vi "SentinelController v33.vi"() -> ()   [LabVIEW 2011] (continued)
                                n2600 = local write "NS6040 tester states H1 hid"(SC_NS6040_tester_states."sending Fullsites?" ("NS6040 tester states H1 hid")) -> ()
                                }
                                frame True {
                                n2601 = flat-sequence {
                                frame #0 {
                                n2602 = while {
                                stop <- w1021 stop-if-true
                                n2603 = Wait (ms)(milliseconds to wait=u32 100) -> ()  [unwired: 1 out]
                                n2604 = One Button Dialog(message="Read error while reading FR?,\nclosing Bus and re-initializing" ("Reply from Sentinel Controller to tester")) -> (true=w1021:bool)  [unwired: 1 in]
                                }
                                }
                                frame #1 {
                                n2605 = local read "VISA bus 1 resource name out hid"() -> (w1027:refnum<visa-resource-name>)
                                n2606 = local read "VISA bus 1 error out hid"() -> (w1026:errorcluster)
                                n2607 = VISA Close(VISA resource name=w1027, error in (no error)=w1026) -> (error out=w1025:errorcluster)
                                n2608 = Unbundle By Name(w1025) -> ("status"=w1024:bool)
                                n2609 = local write "VISA bus 1 close error"(w1024) -> ()
                                }
                                frame #2 {
                                n2610 = local write "VISA bus 1 close error"(FALSE ("H1 online")) -> ()
                                n2611 = local write "NS6040 tester states H1 hid"(SC_NS6040_tester_states."initializing bus" ("NS6040 tester states H1 hid")) -> ()
                                }
                                }
                                }
                                }
                                }
                                frame "sending Fullsites?" {
                                n2612 = flat-sequence {
                                frame #0 {
                                n2613 = flat-sequence {
                                tunnel: [w1035] -> w1032
                                tunnel: [w1034] -> w1030
                                tunnel: [w1041] -> w1033
                                tunnel: w1032 -> [w1041]
                                tunnel: [w1040] -> w1031
                                tunnel: w1030 -> [w1040]
                                tunnel: w1033 -> [w1044]
                                tunnel: w1031 -> [w1043]
                                frame #0 {
                                w1036 = "Fullsites?\n"
                                n2614 = local read "VISA bus 1 resource name out hid"() -> (w1038:refnum<visa-resource-name>)
                                n2615 = local read "VISA bus 1 error out hid"() -> (w1037:errorcluster)
                                n2616 = local write "GPIB bus 1 traffic"(w1036) -> ()
                                n2617 = VISA Write(VISA resource name=w1038, write buffer=w1036, error in (no error)=w1037) -> (VISA resource name out=w1034:refnum<visa-resource-name>, error out=w1035:errorcluster)  [unwired: 1 out]
                                n2618 = Unbundle By Name(w1035) -> ("status"=w1039:bool)
                                n2619 = local write "GPIB bus 1 write error"(w1039) -> ()
                                }
                                frame #1 {
                                n2620 = Wait (ms)(milliseconds to wait=u32 2) -> ()  [unwired: 1 out]
                                }
                                frame #2 {
                                n2621 = local read "GPIB bus 1 traffic"() -> (w1051:string)
                                n2622 = VISA Read(VISA resource name=w1043, byte count=u32 256, error in (no error)=w1044) -> (VISA resource name out=w1046:refnum<visa-resource-name>, read buffer=w1052:string, error out=w1047:errorcluster)  [unwired: 1 out]
                                n2623 = local write "VISA bus 1 resource name out hid"(w1046) -> ()
                                n2624 = local write "H1 FULLSITES? response hid"(w1052) -> ()
                                n2625 = Unbundle By Name(w1047) -> ("status"=w1053:bool)
                                n2626 = Concatenate Strings(w1051, "\r\n", "Bus 1 read: " ("string"), w1052) -> (w1049:string)
                                n2627 = local write "GPIB bus 1 read error"(w1053) -> ()
                                n2628 = local write "GPIB bus 1 traffic"(w1049) -> ()
                                }
                                }
                                }
                                frame #1 {
                                n2629 = local read "GPIB bus 1 read error"() -> (w1054:bool)
                                n2630 = case shown="False" w1054 {
                                frame False {
                                n2631 = flat-sequence {
                                frame #0 {
                                w1063 = "%032b"  # format string
                                n2632 = local read "H1 FULLSITES? response hid"() -> (w1056:string)
                                n2633 = call <vilib>:"Space Constant.vi"() -> ("String"=w1058:string)
                                n2634 = Concatenate Strings("Fullsites" ("regular expression"), w1058) -> (w1057:string)
                                n2635 = call <vilib>:"Trim Whitespace.vi"("string"=w1056) -> ("trimmed string"=w1055:string)  [unwired: 1 in]
                                n2636 = Match Pattern(string=w1055, regular expression=w1057) -> (after substring=w1061:string)  [unwired: 1 in, 3 out]
                                n2637 = Hexadecimal String To Number(string=w1061, default (0uL)=u64 0 ("default (0 U32)")) -> (number=w1064:u64)  [unwired: 1 in, 1 out]
                                n2638 = Format Into String "Format Into String"(format string=w1063, w1064) -> (resulting string=w1060:string)  [unwired: 2 in, 1 out]
                                n2639 = local write "H1 FULLSITES? binary hid"(w1060) -> ()
                                }
                                frame #1 {
                                n2640 = Tick Count (ms)() -> (millisecond timer value=w1068:u32)
                                n2641 = Tick Count (ms)() -> (millisecond timer value=w1067:u32)
                                n2642 = local write "H1 wt start hidden"(w1068) -> ()
                                n2643 = local write "H1 it end hidden"(w1067) -> ()
                                n2644 = local write "H1 Indexing"(FALSE ("h1 indexing")) -> ()
                                n2645 = local write "H1 Testing"(FALSE ("h1 indexing")) -> ()
                                }
                                frame #2 {
                                n2646 = local read "H1 it start hidden"() -> (w1072:u32)
                                n2647 = local read "H1 it end hidden"() -> (w1073:u32)
                                n2648 = Subtract(x=w1073, y=w1072) -> (x-y=w1069:u32)
                                n2649 = Divide(x=w1069, y=u32 1000) -> (x/y=w1071:dbl)
                                n2650 = local write "H1 measured Index Time"(w1071) -> ()
                                }
                                frame #3 {
                                n2651 = local write "NS6040 tester states H1 hid"(SC_NS6040_tester_states."testing" ("NS6040 tester states H1 hid")) -> ()
                                }
                                }
                                }
                                frame True {
                                n2652 = flat-sequence {
                                frame #0 {
                                n2653 = while {
                                stop <- w1075 stop-if-true
                                n2654 = Wait (ms)(milliseconds to wait=u32 100) -> ()  [unwired: 1 out]
                                n2655 = One Button Dialog(message="Read error while reading FULLSITES?,\nclosing Bus and re-initializing" ("Reply from Sentinel Controller to tester")) -> (true=w1075:bool)  [unwired: 1 in]
                                }
                                }
                                frame #1 {
                                n2656 = local read "VISA bus 1 resource name out hid"() -> (w1081:refnum<visa-resource-name>)
                                n2657 = local read "VISA bus 1 error out hid"() -> (w1080:errorcluster)
                                n2658 = VISA Close(VISA resource name=w1081, error in (no error)=w1080) -> (error out=w1079:errorcluster)
                                n2659 = Unbundle By Name(w1079) -> ("status"=w1078:bool)
                                n2660 = local write "VISA bus 1 close error"(w1078) -> ()
                                }
                                frame #2 {
                                n2661 = local write "VISA bus 1 close error"(FALSE ("H1 online")) -> ()
                                n2662 = local write "NS6040 tester states H1 hid"(SC_NS6040_tester_states."initializing bus" ("NS6040 tester states H1 hid")) -> ()
                                }
                                }
                                }
                                }
                                }
                                }
                                }
                                frame "testing" {
                                n2663 = flat-sequence {
                                frame #0 {
                                n2664 = while {
                                stop <- w1084 stop-if-true
                                n2665 = local read "H1 Lock"() -> (w1084:bool)
                                n2666 = Wait (ms)(milliseconds to wait=u32 1) -> ()  [unwired: 1 out]
                                }
                                }
                                frame #1 {
                                n2667 = local write "H1 Ready with sites"(FALSE ("H1 Waiting")) -> ()
                                n2668 = Tick Count (ms)() -> (millisecond timer value=w1095:u32)
                                n2669 = Tick Count (ms)() -> (millisecond timer value=w1094:u32)
                                n2670 = local write "H1 Testing"(TRUE ("testing")) -> ()
                                n2671 = local write "H1 Indexing"(FALSE ("waiting")) -> ()
                                n2672 = local write "H1 wt end hidden"(w1095) -> ()
                                n2673 = local write "H1 tt start hidden"(w1094) -> ()
                                n2674 = local read "GPIB bus 1 traffic"() -> (w1087:string)
                                n2675 = Concatenate Strings(w1087, "\r\n", "Bus 1: " ("string"), "testing" ("string")) -> (w1089:string)
                                n2676 = local write "GPIB bus 1 traffic"(w1089) -> ()
                                }
                                frame #2 {
                                n2677 = local read "H1 wt start hidden"() -> (w1099:u32)
                                n2678 = local read "H1 wt end hidden"() -> (w1100:u32)
                                n2679 = Subtract(x=w1100, y=w1099) -> (x-y=w1098:u32)
                                n2680 = Divide(x=w1098, y=u32 1000) -> (x/y=w1096:dbl)
                                n2681 = local write "H1 measured Wait Time"(w1096) -> ()
                                }
                                frame #3 {
                                n2682 = local write "NS6040 tester states H1 hid"(SC_NS6040_tester_states."sending BINON?" ("NS6040 tester states H1 hid")) -> ()
                                }
                                }
                                }
                                frame "sending BINON?" {
                                n2683 = flat-sequence {
                                tunnel: [w1110] -> w1104
                                tunnel: [w1109] -> w1103
                                tunnel: w1104 -> [w1120]
                                tunnel: w1103 -> [w1119]
                                tunnel: [w1118] -> w1102
                                tunnel: w1102 -> [w1137]
                                frame #0 {
                                n2684 = while {
                                stop <- w1106 continue-if-true
                                n2685 = local read "H1 Lock"() -> (w1106:bool)
                                n2686 = Wait (ms)(milliseconds to wait=u32 1) -> ()  [unwired: 1 out]
                                }
                                }
                                frame #1 {
                                n2687 = local read "Binning string from tester hid"() -> (w1107:string)
                                n2688 = local write "H1 binning string hid"(w1107) -> ()
                                }
                                frame #2 {
                                n2689 = local read "VISA bus 1 resource name out hid"() -> (w1116:refnum<visa-resource-name>)
                                n2690 = local read "VISA bus 1 error out hid"() -> (w1117:errorcluster)
                                n2691 = local read "H1 binning string hid"() -> (w1108:string)
                                n2692 = local read "GPIB bus 1 traffic"() -> (w1114:string)
                                n2693 = VISA Write(VISA resource name=w1116, write buffer=w1108, error in (no error)=w1117) -> (VISA resource name out=w1109:refnum<visa-resource-name>, error out=w1110:errorcluster)  [unwired: 1 out]
                                n2694 = local write "VISA bus 1 error out hid"(w1110) -> ()
                                n2695 = Unbundle By Name(w1110) -> ("status"=w1115:bool)
                                n2696 = Concatenate Strings(w1114, "\r\n", "Bus 1 write: " ("string"), w1108) -> (w1112:string)
                                n2697 = local write "GPIB bus 1 traffic"(w1112) -> ()
                                n2698 = local write "GPIB bus 1 write error"(w1115) -> ()
                                }
                                frame #3 {
                                n2699 = while {
                                tunnel: w1120 -> [w1127]
                                tunnel: w1119 -> [w1126]
                                tunnel: [w1121] -> w1118
                                stop <- w1123 stop-if-true
                                n2700 = local read "GPIB bus 1 traffic"() -> (w1129:string)
                                n2701 = VISA Read(VISA resource name=w1126, byte count=u32 256, error in (no error)=w1127) -> (VISA resource name out=w1134:refnum<visa-resource-name>, read buffer=w1121:string, error out=w1133:errorcluster)  [unwired: 1 out]
                                n2702 = local write "VISA bus 1 resource name out hid"(w1134) -> ()
                                n2703 = Unbundle By Name(w1133) -> ("status"=w1128:bool)
                                n2704 = Match True/False String(2:"false string" ("false string"), 3:"ECHO:", 4:w1121) -> (0:w1123:bool)  [unwired: 1 out]
                                n2705 = local write "GPIB bus 1 read error"(w1128) -> ()
                                n2706 = Concatenate Strings(w1129, "\r\n", "Bus 1 read: " ("string"), w1121) -> (w1131:string)
                                n2707 = local write "GPIB bus 1 traffic"(w1131) -> ()
                                n2708 = Wait (ms)(milliseconds to wait=u32 5) -> ()  [unwired: 1 out]
                                }
                                }
                                frame #4 {
                                n2709 = local read "GPIB bus 1 read error"() -> (w1136:bool)
                                n2710 = case shown="False" w1136 {
                                tunnel: w1137 -> [w1138 _]
                                frame False {
                                n2711 = local write "H1 echo hid"(w1138) -> ()
                                n2712 = local read "H1 binning string hid"() -> (w1139:string)
                                n2713 = Equal?(x=w1138, y=w1139) -> (x = y?=w1140:bool)
                                n2714 = case shown="True" w1140 {
                                frame False {
                                n2715 = local write "NS6040 tester states H1 hid"(SC_NS6040_tester_states."sending ECHONG" ("NS6040 tester states H1 hid")) -> ()
                                }
                                frame True {
                                n2716 = local write "NS6040 tester states H1 hid"(SC_NS6040_tester_states."sending ECHOOK" ("NS6040 tester states H1 hid")) -> ()
                                }
                                }
                                }
                                frame True {
                                n2717 = flat-sequence {
                                frame #0 {
                                n2718 = while {
                                stop <- w1144 stop-if-true
                                n2719 = Wait (ms)(milliseconds to wait=u32 100) -> ()  [unwired: 1 out]
                                n2720 = One Button Dialog(message="Echo readback error for H1.\nClosing Bus 1.", button name ("OK")="Dismiss") -> (true=w1144:bool)
                                }
                                }
                                frame #1 {
                                n2721 = local write "NS6040 tester states H1 hid"(SC_NS6040_tester_states."closing bus" ("NS6040 tester states H1 hid")) -> ()
                                }
                                }
                                }
                                }
                                }
                                }
                                }
                                frame "sending ECHONG" {
                                n2722 = flat-sequence {
                                frame #0 {
                                w1148 = "ECHONG\n"
                                n2723 = local read "VISA bus 1 resource name out hid"() -> (w1155:refnum<visa-resource-name>)
                                n2724 = local read "VISA bus 1 error out hid"() -> (w1156:errorcluster)
                                n2725 = local read "GPIB bus 1 traffic"() -> (w1153:string)
                                n2726 = VISA Write(VISA resource name=w1155, write buffer=w1148, error in (no error)=w1156) -> (error out=w1149:errorcluster)  [unwired: 2 out]
                                n2727 = Unbundle By Name(w1149) -> ("status"=w1154:bool)
                                n2728 = Concatenate Strings(w1153, "\r\n", "Bus 1 write: " ("string"), w1148) -> (w1151:string)
                                n2729 = local write "VISA bus 1 error out hid"(w1149) -> ()
                                n2730 = local write "GPIB bus 1 traffic"(w1151) -> ()
                                n2731 = local write "GPIB bus 1 write error"(w1154) -> ()
                                }
                                frame #1 {
                                n2732 = while {
                                stop <- w1157 stop-if-true
                                n2733 = Wait (ms)(milliseconds to wait=u32 100) -> ()  [unwired: 1 out]
                                n2734 = One Button Dialog(message="ECHO from handler 1 did not match BINON'\nError message from \"sending ECHONG\" state\nBINON message will be resent.") -> (true=w1157:bool)  [unwired: 1 in]
                                }
                                }
                                frame #2 {
                                n2735 = local write "NS6040 tester states H1 hid"(SC_NS6040_tester_states."sending BINON?" ("NS6040 tester states H1 hid")) -> ()
                                }
                                }
                                }
                                frame "sending ECHOOK" {
                                n2736 = flat-sequence {
                                frame #0 {
                                w1161 = "ECHOOK\n"
                                n2737 = local read "VISA bus 1 resource name out hid"() -> (w1168:refnum<visa-resource-name>)
                                n2738 = local read "VISA bus 1 error out hid"() -> (w1169:errorcluster)
                                n2739 = local read "GPIB bus 1 traffic"() -> (w1166:string)
                                n2740 = VISA Write(VISA resource name=w1168, write buffer=w1161, error in (no error)=w1169) -> (error out=w1162:errorcluster)  [unwired: 2 out]
                                n2741 = Unbundle By Name(w1162) -> ("status"=w1167:bool)
                                n2742 = Concatenate Strings(w1166, "\r\n", "Bus 1 write: " ("string"), w1161) -> (w1164:string)
                                n2743 = local write "VISA bus 1 error out hid"(w1162) -> ()
                                n2744 = local write "GPIB bus 1 traffic"(w1164) -> ()
                                n2745 = local write "GPIB bus 1 write error"(w1167) -> ()
                                }
                                frame #1 {
                                n2746 = Tick Count (ms)() -> (millisecond timer value=w1171:u32)
                                n2747 = Tick Count (ms)() -> (millisecond timer value=w1172:u32)
                                n2748 = local write "H1 Ready with sites"(FALSE ("waiting")) -> ()
                                n2749 = local write "H1 Testing"(FALSE ("waiting")) -> ()
                                n2750 = local write "H1 Indexing"(TRUE ("waiting")) -> ()
                                n2751 = local write "H1 tt end hidden"(w1171) -> ()
                                n2752 = local write "H1 it start hidden"(w1172) -> ()
                                }
                                frame #2 {
                                n2753 = local read "H1 tt start hidden"() -> (w1178:u32)
                                n2754 = local read "H1 tt end hidden"() -> (w1179:u32)
                                n2755 = Subtract(x=w1179, y=w1178) -> (x-y=w1177:u32)
                                n2756 = Divide(x=w1177, y=u32 1000) -> (x/y=w1175:dbl)
                                n2757 = local write "H1 measured Test Time"(w1175) -> ()
                                }
                                frame #3 {
                                n2758 = local read "H1 binning string hid"() -> (w1180:string)
                                n2759 = local read "H1 FULLSITES? binary hid"() -> (w1196:string)
                                n2760 = String Subset(string=w1180, offset (0)=6, length (rest)=35 ("length (rest)")) -> (substring=w1192:string)
                                n2761 = local read "H1 Device Count"() -> (w1181:u32)
                                n2762 = local read "H1 Good Units"() -> (w1182:u32)
                                n2763 = Search and Replace String(replace all?=TRUE ("replace all? (F)"), input string=w1192, search string=",") -> (result string=w1186:string)  [unwired: 5 in, 3 out]
                                n2764 = Search and Replace String(replace all?=TRUE ("replace all? (F)"), input string=w1196, search string="1") -> (number of replacements=w1198:i32)  [unwired: 5 in, 3 out]
                                n2765 = Divide(x=w1182, y=w1181) -> (x/y=w1185:dbl)
                                n2766 = Add(x=w1198, y=w1181) -> (x+y=w1197:u32)
                                n2767 = Search and Replace String(replace all?=TRUE ("replace all? (F)"), input string=w1186, search string="1") -> (number of replacements=w1187:i32)  [unwired: 5 in, 3 out]
                                n2768 = local write "H1 Device Count"(w1197) -> ()
                                n2769 = Add(x=w1187, y=w1182) -> (x+y=w1195:u32)
                                n2770 = Multiply(x=w1185, y=100.0) -> (x*y=w1183:dbl)
                                n2771 = local write "H1 Good Units"(w1195) -> ()
                                n2772 = local write "H1 cycle yield hid"(w1183) -> ()
                                }
                                frame #4 {
                                n2773 = local read "H1 Device Count"() -> (w1201:u32)
                                n2774 = local read "H1 Good Units"() -> (w1202:u32)
                                n2775 = Divide(x=w1202, y=w1201) -> (x/y=w1205:dbl)
                                n2776 = Multiply(x=w1205, y=100.0) -> (x*y=w1203:dbl)
                                n2777 = local write "H1 lot yield mon"(w1203) -> ()
                                }
                                frame #5 {
                                n2778 = local write "NS6040 tester states H1 hid"(SC_NS6040_tester_states."serial polling handler" ("NS6040 tester states H1 hid")) -> ()
                                }
                                }
                                }
                                frame "closing bus" {
                                n2779 = local read "GPIB bus 1 traffic"() -> (w1211:string)
                                n2780 = local write "Exit SC tester H1 StMach hid"(TRUE ("Exit H1 state machine hid")) -> ()
                                n2781 = local read "VISA bus 1 resource name out hid"() -> (w1215:refnum<visa-resource-name>)
                                n2782 = local read "VISA bus 1 error out hid"() -> (w1214:errorcluster)
                                n2783 = Concatenate Strings(w1211, "\r\n", "Bus 1: closing " ("string")) -> (w1209:string)
                                n2784 = local write "GPIB bus 1 traffic"(w1209) -> ()
                                n2785 = VISA Close(VISA resource name=w1215, error in (no error)=w1214) -> (error out=w1213:errorcluster)
                                n2786 = Unbundle By Name(w1213) -> ("status"=w1212:bool)
                                n2787 = local write "VISA bus 1 close error"(w1212) -> ()
                                }
                                }
                              }
                              frame #1 {
                                n2788 = local read "Slow for  Diagnostics"() -> (w1216:bool)
                                n2789 = case shown="False" w1216 {
                                frame False {
                                }
                                frame True {
                                n2790 = local read "GPIB wait time (ms)"() -> (w1217:u32)
                                n2791 = Wait (ms)(milliseconds to wait=w1217) -> ()  [unwired: 1 out]
                                }
                                }
                              }
                            }
                            n2792 = local read "Exit SC tester H1 StMach hid"() -> (w903:bool)
                          }
                        }
                      }
                    }
                  }
                }
              }
              n2793 = local read "POWER"() -> (w360:bool)
            }
            n2794 = while {
              stop <- w2197 continue-if-true
              n2795 = local read "H2 online"() -> (w2198:bool)
              n2796 = case shown="True" w2198 {
                frame False {
                }
                frame True {
                  n2797 = flat-sequence {
                    frame #0 {
                      n2798 = local write "Exit SC tester H2 StMach hid"(FALSE ("Exit H2 state machine hid")) -> ()
                    }
                    frame #1 {
                      n2799 = local read "H2 handler type"() -> (w2200:T2)
                      n2800 = case shown="\"Seiko-Epson NS6040\"" w2200 {
                        frame "Multitest" {
                          n2801 = local write "MT99XX tester states H2 hid"(SC_MT99XX_tester_states."initializing bus" ("MT99XX tester states H2 hid")) -> ()
                          n2802 = flat-sequence {
                            frame #0 {
                              n2803 = local read "MT99XX tester states H2 hid"() -> (w2202:T4)
                              n2804 = case shown="\"binning\"" w2202 {
                                frame "initializing bus", Default {
                                n2805 = flat-sequence {
                                frame #0 {
                                # "bus 2"
                                n2806 = local read "GPIB wait timeout hid"() -> (w2205:u32)
                                n2807 = local read "SentCtrl talks to handler 2 at"() -> (w2207:refnum<visa-resource-name>)
                                n2808 = local read "GPIB wait timeout hid"() -> (w2206:u32)
                                n2809 = VISA Open(timeout (0)=w2205, VISA resource name=w2207) -> (VISA resource name=w2204:refnum<visa-resource-name>, error out=w2209:errorcluster)  [unwired: 3 in]
                                n2810 = property class="GPIB Instr"(reference=w2204, error in=w2209, "Timeout"=w2206) -> (error out=w2203:errorcluster)  [unwired: 1 out]
                                n2811 = local write "VISA bus 2 resource name out hid"(w2204) -> ()
                                n2812 = Unbundle By Name(w2203) -> ("status"=w2208:bool)
                                n2813 = local write "VISA bus 2 error out hid"(w2203) -> ()
                                n2814 = local write "VISA bus 2 open error"(w2208) -> ()
                                }
                                frame #1 {
                                n2815 = local write "Exit SC tester H2 StMach hid"(FALSE ("Exit H2 state machine hid")) -> ()
                                n2816 = Concatenate Strings("Bus 2 initializing" ("string"), "\r\n") -> (w2212:string)
                                n2817 = local write "GPIB bus 2 traffic"(w2212) -> ()
                                }
                                frame #2 {
                                n2818 = local write "MT99XX tester states H2 hid"(SC_MT99XX_tester_states."sending *IDN?" ("SC virtual tester states")) -> ()
                                }
                                }
                                }
                                frame "sending *IDN?" {
                                n2819 = flat-sequence {
                                tunnel: [w2224] -> w2217
                                tunnel: [w2223] -> w2216
                                tunnel: w2217 -> [w2238]
                                tunnel: w2216 -> [w2237]
                                tunnel: [w2228] -> w2215
                                tunnel: w2215 -> [w2239]
                                frame #0 {
                                w2218 = "*IDN?"
                                n2820 = local read "VISA bus 2 resource name out hid"() -> (w2227:refnum<visa-resource-name>)
                                n2821 = local read "GPIB bus 2 traffic"() -> (w2222:string)
                                n2822 = local read "VISA bus 2 error out hid"() -> (w2226:errorcluster)
                                n2823 = Concatenate Strings(w2222, "\r\n", "Bus 2 write: " ("string"), w2218) -> (w2220:string)
                                n2824 = VISA Write(VISA resource name=w2227, write buffer=w2218, error in (no error)=w2226) -> (VISA resource name out=w2224:refnum<visa-resource-name>, error out=w2223:errorcluster)  [unwired: 1 out]
                                n2825 = local write "GPIB bus 2 traffic"(w2220) -> ()
                                n2826 = Unbundle By Name(w2223) -> ("status"=w2225:bool)
                                n2827 = local write "GPIB bus 2 write error"(w2225) -> ()
                                }
                                frame #1 {
                                n2828 = local read "GPIB bus 2 traffic"() -> (w2230:string)
                                n2829 = VISA Read(VISA resource name=w2238, byte count=u32 256, error in (no error)=w2237) -> (VISA resource name out=w2235:refnum<visa-resource-name>, read buffer=w2229:string, error out=w2234:errorcluster)  [unwired: 1 out]
                                n2830 = local write "VISA bus 2 resource name out hid"(w2235) -> ()
                                n2831 = Unbundle By Name(w2234) -> ("status"=w2228:bool)
                                n2832 = local write "H2 response to *IDN? hid"(w2229) -> ()
                                n2833 = local write "GPIB bus 2 read error"(w2228) -> ()
                                n2834 = Concatenate Strings(w2230, "\r\n", "Bus 2 read: " ("string"), w2229) -> (w2232:string)
                                n2835 = local write "GPIB bus 2 traffic"(w2232) -> ()
                                }
                                frame #2 {
                                n2836 = case shown="False" w2239 {
                                frame False {
                                n2837 = local write "MT99XX tester states H2 hid"(SC_MT99XX_tester_states."polling *SITES?" ("SC virtual tester states")) -> ()
                                }
                                frame True {
                                n2838 = flat-sequence {
                                frame #0 {
                                n2839 = while {
                                stop <- w2242 stop-if-true
                                n2840 = One Button Dialog(message="Warning:\nVirtual tester does not get a response\nto *IDN? from handler 2.\nCheck GPIB cable and that  handler 2 \nis running and ready to issue a start of test\nby responding with sites ready.", button name ("OK")="Dismiss and retry") -> (true=w2242:bool)
                                n2841 = Wait (ms)(milliseconds to wait=u32 100) -> ()  [unwired: 1 out]
                                }
                                }
                                frame #1 {
                                n2842 = local write "H2 online"(FALSE ("H2 online")) -> ()
                                }
                                frame #2 {
                                n2843 = local write "MT99XX tester states H2 hid"(SC_MT99XX_tester_states."sending *IDN?" ("SC virtual tester states")) -> ()
                                }
                                }
                                }
                                }
                                }
                                }
                                }
                                frame "polling *SITES?" {
                                n2844 = flat-sequence {
                                tunnel: [w2250] -> w2248
                                tunnel: [w2249] -> w2247
                                tunnel: w2248 -> [w2286]
                                tunnel: w2247 -> [w2285]
                                frame #0 {
                                n2845 = while {
                                tunnel: [w2254] -> w2250
                                tunnel: [w2251] -> w2249
                                stop <- w2253 stop-if-true
                                n2846 = stacked-sequence {
                                tunnel: [w2266] -> w2256
                                tunnel: [w2265] -> w2255
                                frame #0 {
                                w2261 = "*SITES?"
                                n2847 = local read "VISA bus 2 resource name out hid"() -> (w2258:refnum<visa-resource-name>)
                                n2848 = local read "VISA bus 2 error out hid"() -> (w2257:errorcluster)
                                n2849 = Concatenate Strings("Handler 2 cycle start" ("string"), "\r\n", "Bus 2 write: " ("string"), w2261) -> (w2263:string)
                                n2850 = VISA Write(VISA resource name=w2258, write buffer=w2261, error in (no error)=w2257) -> (VISA resource name out=w2266:refnum<visa-resource-name>, error out=w2265:errorcluster)  [unwired: 1 out]
                                n2851 = Unbundle By Name(w2265) -> ("status"=w2259:bool)
                                n2852 = local write "GPIB bus 2 traffic"(w2263) -> ()
                                n2853 = local write "GPIB bus 2 write error"(w2259) -> ()
                                }
                                }
                                n2854 = Wait (ms)(milliseconds to wait=u32 1) -> ()  [unwired: 1 out]
                                n2855 = flat-sequence {
                                tunnel: w2256 -> [w2284]
                                tunnel: w2255 -> [w2283]
                                tunnel: [w2270] -> w2254
                                tunnel: [w2268] -> w2253
                                tunnel: [w2267] -> w2251
                                frame #0 {
                                n2856 = local read "GPIB bus 2 traffic"() -> (w2275:string)
                                n2857 = VISA Read(VISA resource name=w2284, byte count=u32 256, error in (no error)=w2283) -> (read buffer=w2270:string, error out=w2281:errorcluster)  [unwired: 2 out]
                                n2858 = Unbundle By Name(w2281) -> ("status"=w2267:bool)
                                n2859 = String Length(string=w2270) -> (length=w2272:i32)
                                n2860 = Scan Value(string=w2270, format string="%b", default (0 dbl)=u8 0) -> (value=w2274:u8)  [unwired: 1 out]
                                n2861 = Concatenate Strings(w2275, "\r\n", "Bus 2 read: " ("string"), w2270) -> (w2277:string)
                                n2862 = local write "GPIB bus 2 read error"(w2267) -> ()
                                n2863 = Greater Than 0?(x=w2272) -> (x > 0?=w2271:bool)
                                n2864 = Greater Than 0?(x=w2274) -> (x > 0?=w2273:bool)
                                n2865 = local write "GPIB bus 2 traffic"(w2277) -> ()
                                n2866 = And(x=w2271, y=w2273) -> (x .and. y?=w2269:bool)
                                n2867 = Or(x=w2269, y=w2267) -> (x .or. y?=w2268:bool)
                                }
                                }
                                }
                                }
                                frame #1 {
                                n2868 = case shown="False" w2285 {
                                tunnel: w2286 -> [w2287 _]
                                frame False {
                                n2869 = flat-sequence {
                                tunnel: w2287 -> [w2288]
                                frame #0 {
                                n2870 = local write "H2 SITES? response hid"(w2288) -> ()
                                n2871 = String Length(string=w2288) -> (length=w2289:i32)
                                n2872 = local write "H2 parallelism"(w2289) -> ()
                                }
                                frame #1 {
                                # "This block adds zeroes (sites not ready)\nto SITES READY from handlers when the\nhandler is running at a lower parallelism\nthan the test program, but has the same\npin mapping for the active sites in common."
                                n2873 = local read "Program Parallelism"() -> (w2291:u32)
                                n2874 = local read "H2 allow lower parallelism"() -> (w2292:bool)
                                n2875 = local read "H2 parallelism"() -> (w2290:u32)
                                n2876 = Less?(x=w2290, y=w2291) -> (x < y?=w2293:bool)
                                n2877 = And(x=w2293, y=w2292) -> (x .and. y?=w2294:bool)
                                n2878 = case shown="False" w2294 {
                                frame False {
                                n2879 = local read "Program Parallelism"() -> (w2297:u32)
                                n2880 = local read "H2 parallelism"() -> (w2295:u32)
                                n2881 = Greater?(x=w2295, y=w2297) -> (0:w2296:bool)
                                n2882 = case shown="True" w2296 {
                                frame False {
                                # "parallelisms must match if arriving here"
                                n2883 = local write "MT99XX tester states H2 hid"(SC_MT99XX_tester_states."testing" ("SC virtual tester states")) -> ()
                                }
                                frame True {
                                n2884 = local write "POWER"(FALSE ("POWER")) -> ()
                                n2885 = local write "MT99XX tester states H2 hid"(SC_MT99XX_tester_states."closing bus" ("SC virtual tester states")) -> ()
                                n2886 = One Button Dialog(message="Fatal error 301:\nTest program cannot support higher\nparallelism on handler 2.\nThe Sentinel Controller program is shutting down.\nPlease correct the mismatch and restart.") -> ()  [unwired: 1 in, 1 out]
                                }
                                }
                                }
                                frame True {
                                n2887 = local read "Program Parallelism"() -> (w2307:u32)
                                n2888 = local read "H2 parallelism"() -> (w2305:u32)
                                n2889 = local read "H2 SITES? response hid"() -> (w2303:string)
                                n2890 = local write "MT99XX tester states H2 hid"(SC_MT99XX_tester_states."testing" ("SC virtual tester states")) -> ()
                                n2891 = Subtract(x=w2307, y=w2305) -> (x-y=w2306:u32)
                                n2892 = for {
                                N: w2306 -> [_]
                                shift-right: [w2308] -> w2302
                                shift-left: w2303 -> [w2309]
                                n2893 = Concatenate Strings(w2309, "0" ("string")) -> (w2308:string)
                                }
                                n2894 = local write "H2 SITES? response hid"(w2302) -> ()
                                }
                                }
                                }
                                frame #2 {
                                n2895 = Tick Count (ms)() -> (millisecond timer value=w2315:u32)
                                n2896 = Tick Count (ms)() -> (millisecond timer value=w2314:u32)
                                n2897 = local write "H2 Ready with sites"(TRUE ("H2 Waiting")) -> ()
                                n2898 = local write "H2 Indexing"(FALSE ("h1 indexing")) -> ()
                                n2899 = local write "H2 Testing"(FALSE ("h1 indexing")) -> ()
                                n2900 = local write "H2 wt start hidden"(w2315) -> ()
                                n2901 = local write "H2 it end hidden"(w2314) -> ()
                                }
                                frame #3 {
                                n2902 = local read "H2 it start hidden"() -> (w2319:u32)
                                n2903 = local read "H2 it end hidden"() -> (w2320:u32)
                                n2904 = Subtract(x=w2320, y=w2319) -> (x-y=w2316:u32)
                                n2905 = local write "MT99XX tester states H2 hid"(SC_MT99XX_tester_states."testing" ("SC virtual tester states")) -> ()
                                n2906 = Divide(x=w2316, y=u32 1000) -> (x/y=w2318:dbl)
                                n2907 = local write "H2 measured  Index Time"(w2318) -> ()
                                }
                                }
                                }
                                frame True {
                                n2908 = flat-sequence {
                                frame #0 {
                                n2909 = local read "VISA bus 2 resource name out hid"() -> (w2325:refnum<visa-resource-name>)
                                n2910 = local read "VISA bus 2 error out hid"() -> (w2324:errorcluster)
                                n2911 = VISA Close(VISA resource name=w2325, error in (no error)=w2324) -> (error out=w2323:errorcluster)
                                n2912 = Unbundle By Name(w2323) -> ("status"=w2322:bool)
                                n2913 = local write "VISA bus 2 close error"(w2322) -> ()
                                }
                                frame #1 {
                                n2914 = local write "VISA bus 2 close error"(FALSE ("VISA bus 1 close error")) -> ()
                                n2915 = Concatenate Strings("Bus 2 error  while reading,\nclosing Bus 2 and re-initializing" ("string"), "\r\n") -> (w2327:string)
                                n2916 = local write "GPIB bus 2 traffic"(w2327) -> ()
                                }
                                frame #2 {
                                n2917 = local write "MT99XX tester states H2 hid"(SC_MT99XX_tester_states."initializing bus" ("SC virtual tester states")) -> ()
                                }
                                }
                                }
                                }
                                }
                                }
                                }
                                frame "testing" {
                                n2918 = flat-sequence {
                                frame #0 {
                                n2919 = while {
                                stop <- w2331 stop-if-true
                                n2920 = local read "H2 Lock"() -> (w2331:bool)
                                n2921 = Wait (ms)(milliseconds to wait=u32 1) -> ()  [unwired: 1 out]
                                }
                                }
                                frame #1 {
                                n2922 = Tick Count (ms)() -> (millisecond timer value=w2343:u32)
                                n2923 = Tick Count (ms)() -> (millisecond timer value=w2342:u32)
                                n2924 = local write "H2 Ready with sites"(FALSE ("waiting")) -> ()
                                n2925 = local write "H2 Indexing"(FALSE ("waiting")) -> ()
                                n2926 = local write "H2 Testing"(TRUE ("testing")) -> ()
                                n2927 = local write "H2 wt end hidden"(w2343) -> ()
                                n2928 = local write "H2 tt start hidden"(w2342) -> ()
                                n2929 = local read "GPIB bus 2 traffic"() -> (w2334:string)
                                n2930 = local write "MT99XX tester states H2 hid"(SC_MT99XX_tester_states."binning" ("SC virtual tester states")) -> ()
                                n2931 = Concatenate Strings(w2334, "\r\n", "Bus 2: " ("string"), "testing" ("string")) -> (w2336:string)
                                n2932 = local write "GPIB bus 2 traffic"(w2336) -> ()
                                }
                                frame #2 {
                                n2933 = local read "H2 wt start hidden"() -> (w2345:u32)
                                n2934 = local read "H2 wt end hidden"() -> (w2344:u32)
                                n2935 = Subtract(x=w2344, y=w2345) -> (x-y=w2348:u32)
                                n2936 = Divide(x=w2348, y=u32 1000) -> (x/y=w2346:dbl)
                                n2937 = local write "H2 measured Wait Time"(w2346) -> ()
                                }
                                frame #3 {
                                n2938 = local write "MT99XX tester states H2 hid"(SC_MT99XX_tester_states."binning" ("MT99XX tester states H2 hid")) -> ()
                                }
                                }
                                }
                                frame "binning" {
                                n2939 = flat-sequence {
                                tunnel: [w2361] -> w2352
                                tunnel: [w2388] -> w2353
                                tunnel: w2352 -> [w2388]
                                tunnel: w2353 -> [w2395]
                                tunnel: [w2394] -> w2351
                                tunnel: [w2393] -> w2350
                                tunnel: w2351 -> [w2446]
                                tunnel: w2350 -> [w2445]
                                frame #0 {
                                n2940 = while {
                                stop <- w2355 continue-if-true
                                n2941 = local read "H2 Lock"() -> (w2355:bool)
                                n2942 = Wait (ms)(milliseconds to wait=u32 1) -> ()  [unwired: 1 out]
                                }
                                }
                                frame #1 {
                                n2943 = local read "Program Parallelism"() -> (w2358:u32)
                                n2944 = local read "H2 parallelism"() -> (w2357:u32)
                                n2945 = local read "H2 allow lower parallelism"() -> (w2359:bool)
                                n2946 = Less?(x=w2357, y=w2358) -> (x < y?=w2360:bool)
                                n2947 = And(x=w2360, y=w2359) -> (x .and. y?=w2356:bool)
                                n2948 = case shown="True" w2356 {
                                tunnel: [w2362 w2373] -> w2361
                                frame False {
                                n2949 = local read "VISA bus 2 resource name out hid"() -> (w2370:refnum<visa-resource-name>)
                                n2950 = local read "Binning string from tester hid"() -> (w2362:string)
                                n2951 = local read "VISA bus 2 error out hid"() -> (w2371:errorcluster)
                                n2952 = local read "GPIB bus 2 traffic"() -> (w2366:string)
                                n2953 = VISA Write(VISA resource name=w2370, write buffer=w2362, error in (no error)=w2371) -> (VISA resource name out=w2368:refnum<visa-resource-name>, error out=w2369:errorcluster)  [unwired: 1 out]
                                n2954 = local write "VISA bus 2 resource name out hid"(w2368) -> ()
                                n2955 = local write "VISA bus 2 error out hid"(w2369) -> ()
                                n2956 = Unbundle By Name(w2369) -> ("status"=w2367:bool)
                                n2957 = Concatenate Strings(w2366, "\r\n", "Bus 2 write: " ("string"), w2362) -> (w2364:string)
                                n2958 = local write "GPIB bus 2 write error"(w2367) -> ()
                                n2959 = local write "GPIB bus 2 traffic"(w2364) -> ()
                                }
                                frame True {
                                n2960 = local read "H2 parallelism"() -> (w2372:u32)
                                n2961 = local read "Binning string from tester hid"() -> (w2374:string)
                                n2962 = local read "VISA bus 2 resource name out hid"() -> (w2385:refnum<visa-resource-name>)
                                n2963 = Multiply(x=w2372, y=u32 8) -> (x*y=w2376:u32)
                                n2964 = local read "VISA bus 2 error out hid"() -> (w2386:errorcluster)
                                n2965 = local read "GPIB bus 2 traffic"() -> (w2381:string)
                                n2966 = Decrement(x=w2376) -> (x-1=w2377:u32)
                                n2967 = String Subset(string=w2374, length (rest)=w2377) -> (substring=w2373:string)  [unwired: 1 in]
                                n2968 = VISA Write(VISA resource name=w2385, write buffer=w2373, error in (no error)=w2386) -> (VISA resource name out=w2383:refnum<visa-resource-name>, error out=w2384:errorcluster)  [unwired: 1 out]
                                n2969 = local write "VISA bus 2 resource name out hid"(w2383) -> ()
                                n2970 = local write "VISA bus 2 error out hid"(w2384) -> ()
                                n2971 = Unbundle By Name(w2384) -> ("status"=w2382:bool)
                                n2972 = Concatenate Strings(w2381, "\r\n", "Bus 2 write: " ("string"), w2373) -> (w2379:string)
                                n2973 = local write "GPIB bus 2 traffic"(w2379) -> ()
                                n2974 = local write "GPIB bus 2 write error"(w2382) -> ()
                                }
                                }
                                }
                                frame #2 {
                                n2975 = Tick Count (ms)() -> (millisecond timer value=w2390:u32)
                                n2976 = Tick Count (ms)() -> (millisecond timer value=w2389:u32)
                                n2977 = local write "H2 Ready with sites"(FALSE ("waiting")) -> ()
                                n2978 = local write "H2 Testing"(FALSE ("waiting")) -> ()
                                n2979 = local write "H2 Indexing"(TRUE ("waiting")) -> ()
                                n2980 = local write "H2 it start hidden"(w2390) -> ()
                                n2981 = local write "H2 tt end hidden"(w2389) -> ()
                                }
                                frame #3 {
                                n2982 = while {
                                tunnel: [w2418] -> w2414 mode=indexing
                                shift-right: [w2419] -> _
                                shift-left: w2395 -> [w2421]
                                stop <- w2416 stop-if-true
                                n2983 = Match Pattern(string=w2421, regular expression=" ") -> (before substring=w2418:string, after substring=w2419:string, offset past match=w2417:i32)  [unwired: 2 out]
                                n2984 = Less Than 0?(x=w2417) -> (x < 0?=w2416:bool)
                                }
                                n2985 = local read "H2 tt start hidden"() -> (w2399:u32)
                                n2986 = local read "H2 tt end hidden"() -> (w2400:u32)
                                n2987 = Subtract(x=w2400, y=w2399) -> (x-y=w2398:u32)
                                n2988 = Divide(x=w2398, y=u32 1000) -> (x/y=w2396:dbl)
                                n2989 = Array Size(array=w2414) -> (size(s)=w2411:i32)
                                n2990 = local read "H2 SITES? response hid"() -> (w2406:string)
                                n2991 = local read "H2 parallelism"() -> (w2405:u32)
                                n2992 = local write "H2 measured Test Time"(w2396) -> ()
                                n2993 = Divide(x=w2411, y=3) -> (x/y=w2413:dbl)
                                n2994 = To Unsigned Byte Integer(number=w2413) -> (unsigned 8bit integer=w2409:u8)
                                n2995 = Not Equal?(x=w2405, y=w2409) -> (x != y?=w2410:bool)
                                n2996 = case shown="True" w2410 {
                                frame False {
                                }
                                frame True {
                                n2997 = One Button Dialog(message="Warning:\nH2 Parallelism Mismatch!\nEither allow this from the system configuration tab\nor change the parallelism on H2. This message will\ncontinue until the problem is corrected.") -> ()  [unwired: 1 in, 1 out]
                                }
                                }
                                n2998 = for {
                                N: w2409 -> [_]
                                tunnel: w2414 -> [w2444]
                                tunnel: w2406 -> [w2435]
                                shift-right: [w2428] -> w2393
                                shift-left: 0 -> [w2427]
                                shift-right: [w2424] -> w2394
                                shift-left: 0 -> [w2422]
                                i -> [w2425]
                                n2999 = Increment(x=w2422) -> (x+1=w2423:i32)
                                n3000 = Increment(x=w2427) -> (x+1=w2426:i32)
                                n3001 = Increment(x=w2425) -> (x+1=w2443:i32)
                                n3002 = String Subset(string=w2435, offset (0)=w2425, length (rest)=1 ("length (rest)")) -> (substring=w2431:string)
                                n3003 = Multiply(x=3, y=w2443) -> (x*y=w2437:i32)
                                n3004 = Equal?(x=w2431, y="1") -> (x = y?=w2429:bool)
                                n3005 = Select(t=w2426, s=w2429, f=w2427) -> (s? t:f=w2428:i32)
                                n3006 = Decrement(x=w2437) -> (x-1=w2436:i32)
                                n3007 = Index Array(array=w2444, index=w2436) -> (element=w2441:string)
                                n3008 = Decimal String To Number(string=w2441, offset=0) -> (number=w2439:i32)  [unwired: 1 in, 1 out]
                                n3009 = Equal?(x=w2439, y=1) -> (x = y?=w2432:bool)
                                n3010 = And(x=w2432, y=w2429) -> (x .and. y?=w2433:bool)
                                n3011 = Select(t=w2423, s=w2433, f=w2422) -> (s? t:f=w2424:i32)
                                }
                                n3012 = local read "H2 Device Count"() -> (w2402:u32)
                                n3013 = local read "H2 Good Units"() -> (w2403:u32)
                                n3014 = Add(x=w2403, y=w2394) -> (x+y=w2404:u32)
                                n3015 = Add(x=w2402, y=w2393) -> (x+y=w2401:u32)
                                n3016 = local write "H2 Good Units"(w2404) -> ()
                                n3017 = local write "H2 Device Count"(w2401) -> ()
                                }
                                frame #4 {
                                n3018 = Divide(x=w2446, y=w2445) -> (x/y=w2447:dbl)
                                n3019 = local read "H2 Device Count"() -> (w2450:u32)
                                n3020 = local read "H2 Good Units"() -> (w2451:u32)
                                n3021 = Multiply(x=w2447, y=100.0) -> (x*y=w2449:dbl)
                                n3022 = local write "H2 cycle yield hid"(w2449) -> ()
                                n3023 = Divide(x=w2451, y=w2450) -> (x/y=w2454:dbl)
                                n3024 = Multiply(x=w2454, y=100.0) -> (x*y=w2452:dbl)
                                n3025 = local write "H2 lot yield mon"(w2452) -> ()
                                }
                                frame #5 {
                                n3026 = local read "H2 online"() -> (w2455:bool)
                                n3027 = local read "POWER"() -> (w2457:bool)
                                n3028 = Compound Arithmetic op=AND(w2455, w2457) -> (w2456:bool)
                                n3029 = case shown="False" w2456 {
                                frame False {
                                n3030 = local write "MT99XX tester states H2 hid"(SC_MT99XX_tester_states."closing bus" ("SC virtual tester states")) -> ()
                                }
                                frame True {
                                n3031 = local write "MT99XX tester states H2 hid"(SC_MT99XX_tester_states."polling *SITES?" ("SC virtual tester states")) -> ()
                                }
                                }
                                }
                                }
                                }
                                frame "closing bus" {
                                n3032 = local read "GPIB bus 2 traffic"() -> (w2464:string)
                                n3033 = local write "Exit SC tester H2 StMach hid"(TRUE ("Exit H2 state machine hid")) -> ()
                                n3034 = local read "VISA bus 2 resource name out hid"() -> (w2468:refnum<visa-resource-name>)
                                n3035 = local read "VISA bus 2 error out hid"() -> (w2467:errorcluster)
                                n3036 = Concatenate Strings(w2464, "\r\n", "Bus 2: closing " ("string")) -> (w2462:string)
                                n3037 = local write "GPIB bus 2 traffic"(w2462) -> ()
                                n3038 = VISA Close(VISA resource name=w2468, error in (no error)=w2467) -> (error out=w2466:errorcluster)
                                n3039 = Unbundle By Name(w2466) -> ("status"=w2465:bool)
                                n3040 = local write "VISA bus 2 close error"(w2465) -> ()
                                }
                              }
                            }
                            frame #1 {
                              n3041 = local read "Slow for  Diagnostics"() -> (w2469:bool)
                              n3042 = case shown="True" w2469 {
                                frame False {
                                }
                                frame True {
                                n3043 = local read "GPIB wait time (ms)"() -> (w2470:u32)
                                n3044 = Wait (ms)(milliseconds to wait=w2470) -> ()  [unwired: 1 out]
                                }
                              }
                            }
                          }
                        }
                        frame "DeltaDesign" {
                          n3045 = local write "MT99XX tester states H2 hid"(SC_MT99XX_tester_states."initializing bus" ("MT99XX tester states H2 hid")) -> ()
                          n3046 = flat-sequence {
                            frame #0 {
                              n3047 = local read "MT99XX tester states H2 hid"() -> (w2472:T4)
                              n3048 = case shown="\"binning\"" w2472 {
                                frame "initializing bus", Default {
                                n3049 = flat-sequence {
                                frame #0 {
                                # "bus 2"
                                n3050 = local read "GPIB wait timeout hid"() -> (w2475:u32)
                                n3051 = local read "SentCtrl talks to handler 2 at"() -> (w2477:refnum<visa-resource-name>)
